vi "发送open.vi"(7 "Message Priority (Normal)":T2=enum."Normal" caption="消息优先级（标准）", 8 "error in (no error)":errorcluster caption="错误输入（无错误）", 10 "input":T1, 11 "Message Enqueuer":refnum<class "Message Enqueuer.lvclass"> caption="消息待入队列") -> (0 "error out":errorcluster caption="错误输出", 3 "Message Enqueuer out":refnum<class "Message Enqueuer.lvclass"> caption="消息待入队列输出")   [LabVIEW 2016, in "数据传输系统-03.lvlib" / "update.lvlib" / "open消息.lvclass"]
doc: "本VI将消息发送至操作者。"
uses:
  <vilib>/ActorFramework/Message Enqueuer/Message Enqueuer.lvclass
  <vilib>/ActorFramework/Message Enqueuer/Message Priority.ctl
  C:/Program Files (x86)/National Instruments/LabVIEW 2016/vi.lib/ActorFramework/Message/Message.lvclass
  <vilib>/ActorFramework/Message Enqueuer/Message Enqueuer.lvclass/Message Enqueuer.ctl
  <vilib>/ActorFramework/Message Priority Queue/Priority Enqueue.vi
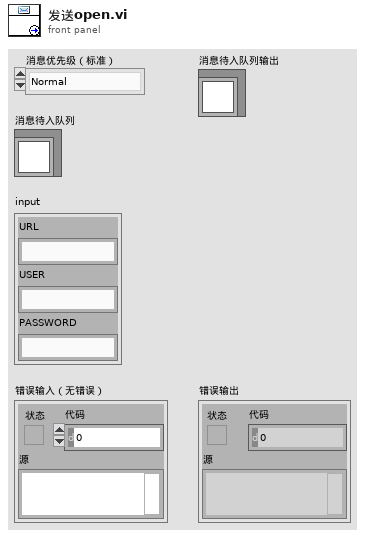
[diagram p1: front panel]
types:
  T1 = cluster{"URL":string, "USER":string, "PASSWORD":string}
  T2 = typedef "Actor Framework.lvlib/Message Enqueuer.lvclass/Message Priority.ctl" = enum16{"Low", "Normal", "High"}
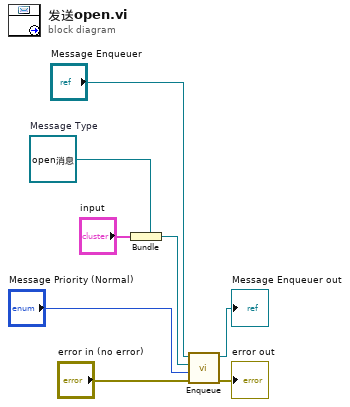
[diagram p0: block diagram]
diagram:
  w5 = refnum<class "open消息.lvclass"> refnum  # Message Type
  n1 = Bundle(cluster=w5, "input") -> (w4:refnum<class "open消息.lvclass">)
  n2 = call <vilib>:"Enqueue.vi"("error in (no error)"="error in (no error)", "Message Priority (Normal)"="Message Priority (Normal)", "Message"=w4, "Message Enqueuer in"="Message Enqueuer") -> ("error out"=→"error out":errorcluster, "Message Enqueuer out"=→"Message Enqueuer out":refnum<class "Message Enqueuer.lvclass">)  [unwired: 6 in]
